vi "Func-엑셀 데이터를 그래프로 출력.vi"() -> ()   [LabVIEW 2015] (continued)
-19.24\t-17.452\n-18.3\t-19.24\t-17.442\n-18.3\t-19.23\t-17.435\n-18.3\t-19.22\t-17.427\n-18.3\t-19.22\t-17.422\n-18.3\t-19.22\t-17.417\n-18.3\t-19.21\t-17.409\n-18.3\t-19.21\t-17.403\n-18.3\t-19.2\t-17.397\n-18.3\t-19.2\t-17.384\n-18.3\t-19.19\t-17.38\n-18.3\t-19.18\t-17.376\n-18.3\t-19.17\t-17.365\n-18.3\t-19.17\t-17.361\n-18.3\t-19.16\t-17.356\n-18.3\t-19.15\t-17.347\n-18.3\t-19.15\t-17.342\n-18.3\t-19.14\t-17.333\n-18.3\t-19.14\t-17.326\n-18.3\t-19.14\t-17.316\n-18.3\t-19.14\t-17.306\n-18.3\t-19.13\t-17.302\n-18.3\t-19.12\t-17.293\n-18.3\t-19.12\t-17.285\n-18.3\t-19.11\t-17.277\n-18.3\t-19.1\t-17.278\n-18.3\t-19.1\t-17.273\n-18.3\t-19.09\t-17.261\n-18.3\t-19.08\t-17.253\n-18.3\t-19.08\t-17.249\n-18.3\t-19.07\t-17.241\n-18.3\t-19.07\t-17.228\n-18.3\t-19.06\t-17.219\n-18.3\t-19.06\t-17.211\n-18.3\t-19.05\t-17.209\n-18.3\t-19.05\t-17.198\n-18.3\t-19.04\t-17.191\n-18.3\t-19.04\t-17.187\n-18.3\t-19.03\t-17.183\n-18.3\t-19.03\t-17.173\n-18.3\t-19.02\t-17.164\n-18.3\t-19.01\t-17.159\n-18.3\t-19\t-17.15\n-18.3\t-19\t-17.142\n-18.3\t-18.99\t-17.134\n-18.3\t-18.99\t-17.129\n-18.3\t-18.99\t-17.123\n-18.3\t-18.99\t-17.114\n-18.3\t-18.98\t-17.109\n-18.3\t-18.97\t-17.102\n-18.3\t-18.97\t-17.091\n-18.3\t-18.96\t-17.084\n-18.3\t-18.95\t-17.078\n-18.3\t-18.94\t-17.068\n-18.3\t-18.94\t-17.059\n-18.3\t-18.93\t-17.053\n-18.3\t-18.93\t-17.047\n-18.3\t-18.92\t-17.04\n-18.3\t-18.92\t-17.032\n-18.3\t-18.91\t-17.025\n-18.3\t-18.91\t-17.02\n-18.3\t-18.9\t-17.014\n-18.3\t-18.9\t-17.006\n-18.3\t-18.9\t-16.998\n-18.3\t-18.9\t-16.993\n-18.3\t-18.9\t-16.983\n-18.3\t-18.89\t-16.98\n-18.3\t-18.88\t-16.971\n-18.3\t-18.87\t-16.957\n-18.3\t-18.86\t-16.95\n-18.3\t-18.86\t-16.944\n-18.3\t-18.85\t-16.934\n-18.3\t-18.84\t-16.927\n-18.3\t-18.84\t-16.92\n-18.3\t-18.84\t-16.914\n-18.3\t-18.83\t-16.914\n-18.3\t-18.83\t-16.905\n-18.3\t-18.82\t-16.9\n-18.3\t-18.82\t-16.891\n-18.3\t-18.82\t-16.887\n-18.3\t-18.81\t-16.88\n-18.3\t-18.81\t-16.871\n-18.3\t-18.8\t-16.868\n-18.3\t-18.79\t-16.857\n-18.3\t-18.79\t-16.852\n-18.3\t-18.78\t-16.845\n-18.3\t-18.78\t-16.832\n-18.3\t-18.77\t-16.824\n-18.3\t-18.76\t-16.816\n-18.3\t-18.76\t-16.809\n-18.3\t-18.75\t-16.799\n-18.3\t-18.75\t-16.791\n-18.3\t-18.75\t-16.782\n-18.3\t-18.75\t-16.776\n-18.3\t-18.74\t-16.77\n-18.3\t-18.74\t-16.761\n-18.3\t-18.74\t-16.76\n-18.3\t-18.73\t-16.756\n-18.3\t-18.72\t-16.75\n-18.3\t-18.72\t-16.744\n-18.3\t-18.71\t-16.736\n-18.3\t-18.71\t-16.73\n-18.3\t-18.7\t-16.721\n-18.3\t-18.7\t-16.713\n-18.3\t-18.69\t-16.701\n-18.3\t-18.69\t-16.693\n-18.3\t-18.68\t-16.687\n-18.3\t-18.68\t-16.675\n-18.3\t-18.67\t-16.67\n-18.3\t-18.67\t-16.664\n-18.3\t-18.67\t-16.659\n-18.3\t-18.67\t-16.653\n-18.3\t-18.66\t-16.642\n-18.3\t-18.65\t-16.634\n-18.3\t-18.65\t-16.629\n-18.3\t-18.65\t-16.62\n-18.3\t-18.64\t-16.617\n-18.3\t-18.64\t-16.611\n-18.3\t-18.63\t-16.607\n-18.3\t-18.63\t-16.601\n-18.3\t-18.62\t-16.595\n-18.3\t-18.62\t-16.587\n-18.3\t-18.62\t-16.576\n-18.3\t-18.61\t-16.569\n-18.3\t-18.61\t-16.559\n-18.3\t-18.6\t-16.552\n-18.3\t-18.6\t-16.545\n-18.3\t-18.59\t-16.534\n-18.3\t-18.59\t-16.529\n-18.3\t-18.59\t-16.523\n-18.3\t-18.59\t-16.516\n-18.3\t-18.59\t-16.508\n-18.3\t-18.59\t-16.5\n-18.3\t-18.59\t-16.493\n-18.3\t-18.58\t-16.486\n-18.3\t-18.58\t-16.478\n-18.3\t-18.58\t-16.467\n-18.3\t-18.57\t-16.461\n-18.3\t-18.56\t-16.454\n-18.3\t-18.56\t-16.446\n-18.3\t-18.55\t-16.439\n-18.3\t-18.55\t-16.431\n-18.3\t-18.54\t-16.424\n-18.3\t-18.55\t-16.419\n-18.3\t-18.54\t-16.414\n-18.3\t-18.54\t-16.404\n-18.3\t-18.53\t-16.398\n-18.3\t-18.53\t-16.395\n-18.3\t-18.53\t-16.384\n-18.3\t-18.52\t-16.379\n-18.3\t-18.52\t-16.375\n-18.3\t-18.51\t-16.366\n-18.3\t-18.51\t-16.358\n-18.3\t-18.51\t-16.35\n-18.3\t-18.51\t-16.344\n-18.3\t-18.51\t-16.331\n-18.3\t-18.51\t-16.322\n-18.3\t-18.5\t-16.316\n-18.3\t-18.5\t-16.311\n-18.3\t-18.49\t-16.304\n-18.3\t-18.49\t-16.295\n-18.3\t-18.49\t-16.293\n-18.3\t-18.49\t-16.288\n-18.3\t-18.49\t-16.28\n-18.3\t-18.49\t-16.274\n-18.3\t-18.48\t-16.265\n-18.3\t-18.48\t-16.261\n-18.3\t-18.48\t-16.254\n-18.3\t-18.48\t-16.252\n-18.3\t-18.47\t-16.242\n-18.3\t-18.47\t-16.233\n-18.3\t-18.47\t-16.224\n-18.3\t-18.46\t-16.216\n-18.3\t-18.46\t-16.209\n-18.3\t-18.46\t-16.196\n-18.3\t-18.46\t-16.188\n-18.3\t-18.45\t-16.184\n-18.3\t-18.45\t-16.177\n-18.3\t-18.45\t-16.17\n-18.3\t-18.44\t-16.164\n-18.3\t-18.44\t-16.156\n-18.3\t-18.44\t-16.149\n-18.3\t-18.44\t-16.143\n-18.3\t-18.44\t-16.132\n-18.3\t-18.44\t-16.127\n-18.3\t-18.43\t-16.121\n-18.3\t-18.43\t-16.108\n-18.3\t-18.43\t-16.102\n-18.3\t-18.43\t-16.096\n-18.3\t-18.43\t-16.089\n-18.3\t-18.43\t-16.082\n-18.3\t-18.42\t-16.074\n-18.3\t-18.42\t-16.071\n-18.3\t-18.42\t-16.064\n-18.3\t-18.42\t-16.057\n-18.3\t-18.42\t-16.052\n-18.3\t-18.42\t-16.048\n-18.3\t-18.41\t-16.043\n-18.3\t-18.4\t-16.033\n-18.3\t-18.4\t-16.026\n-18.3\t-18.4\t-16.021\n-18.3\t-18.4\t-16.01\n-18.3\t-18.4\t-16.004\n-18.3\t-18.4\t-15.996\n-18.3\t-18.4\t-15.989\n-18.3\t-18.39\t-15.983\n-18.3\t-18.39\t-15.971\n-18.3\t-18.39\t-15.962\n-18.3\t-18.39\t-15.952\n-18.3\t-18.39\t-15.949\n-18.3\t-18.39\t-15.94\n-18.3\t-18.38\t-15.936\n-18.3\t-18.38\t-15.929\n-18.3\t-18.38\t-15.921\n-18.3\t-18.37\t-15.916\n-18.3\t-18.37\t-15.909\n-18.3\t-18.37\t-15.898\n-18.3\t-18.37\t-15.892\n-18.3\t-18.37\t-15.883\n-18.3\t-18.37\t-15.876\n-18.3\t-18.37\t-15.868\n-18.3\t-18.36\t-15.858\n-18.3\t-18.36\t-15.85\n-18.3\t-18.36\t-15.841\n-18.3\t-18.36\t-15.837\n-18.3\t-18.35\t-15.831\n-18.3\t-18.35\t-15.83\n-18.3\t-18.35\t-15.822\n-18.3\t-18.35\t-15.817\n-18.3\t-18.35\t-15.812\n-18.3\t-18.35\t-15.798\n-18.3\t-18.35\t-15.792\n-18.3\t-18.35\t-15.785\n-18.3\t-18.34\t-15.777\n-18.3\t-18.34\t-15.769\n-18.3\t-18.34\t-15.763\n-18.3\t-18.34\t-15.759\n-18.3\t-18.34\t-15.752\n-18.3\t-18.33\t-15.743\n-18.3\t-18.34\t-15.735\n-18.3\t-18.33\t-15.73\n-18.3\t-18.33\t-15.723\n-18.3\t-18.33\t-15.712\n-18.3\t-18.33\t-15.707\n-18.3\t-18.33\t-15.702\n-18.3\t-18.33\t-15.695\n-18.3\t-18.33\t-15.688\n-18.3\t-18.32\t-15.685\n-18.3\t-18.32\t-15.679\n-18.3\t-18.31\t-15.67\n-18.3\t-18.31\t-15.661\n-18.3\t-18.31\t-15.653\n-18.3\t-18.31\t-15.646\n-18.3\t-18.31\t-15.639\n-18.3\t-18.31\t-15.632\n-18.3\t-18.31\t-15.63\n-18.3\t-18.31\t-15.626\n-18.3\t-18.31\t-15.619\n-18.3\t-18.31\t-15.614\n-18.3\t-18.31\t-15.607\n-18.3\t-18.31\t-15.598\n-18.3\t-18.31\t-15.589\n-18.3\t-18.31\t-15.583\n-18.3\t-18.31\t-15.57\n-18.3\t-18.31\t-15.561\n-18.3\t-18.31\t-15.553\n-18.3\t-18.31\t-15.548\n-18.3\t-18.31\t-15.544\n-18.3\t-18.31\t-15.533\n-18.3\t-18.31\t-15.533\n-18.3\t-18.31\t-15.53\n-18.3\t-18.31\t-15.518\n-18.3\t-18.31\t-15.512\n-18.3\t-18.31\t-15.504\n-18.3\t-18.31\t-15.493\n-18.3\t-18.31\t-15.485\n-18.3\t-18.31\t-15.477\n-18.3\t-18.31\t-15.467\n-18.3\t-18.31\t-15.463\n-18.3\t-18.31\t-15.458\n-18.3\t-18.31\t-15.457\n-18.3\t-18.31\t-15.448\n-18.3\t-18.31\t-15.441\n-18.3\t-18.31\t-15.433\n-18.3\t-18.31\t-15.428\n-18.3\t-18.31\t-15.422\n-18.3\t-18.31\t-15.411\n-18.3\t-18.31\t-15.407\n-18.3\t-18.31\t-15.402\n-18.3\t-18.31\t-15.395\n-18.3\t-18.31\t-15.386\n-18.3\t-18.31\t-15.38\n-18.3\t-18.31\t-15.369\n-18.3\t-18.31\t-15.359\n-18.3\t-18.31\t-15.352\n-18.3\t-18.31\t-15.343\n-18.3\t-18.31\t-15.337\n-18.3\t-18.31\t-15.33\n-18.3\t-18.31\t-15.323\n-18.3\t-18.31\t-15.32\n-18.3\t-18.29\t-15.314\n-18.3\t-18.29\t-15.307\n-18.3\t-18.29\t-15.302\n-18.3\t-18.29\t-15.293\n-18.3\t-18.29\t-15.288\n-18.3\t-18.29\t-15.279\n-18.3\t-18.29\t-15.274\n-18.3\t-18.29\t-15.266\n-18.3\t-18.29\t-15.264\n-18.3\t-18.29\t-15.257\n-18.3\t-18.29\t-15.25\n-18.3\t-18.29\t-15.243\n-18.3\t-18.29\t-15.238\n-18.3\t-18.29\t-15.228\n-18.3\t-18.29\t-15.221\n-18.3\t-18.29\t-15.216\n-18.3\t-18.29\t-15.206\n-18.3\t-18.29\t-15.203\n-18.3\t-18.29\t-15.193\n-18.3\t-18.28\t-15.185\n-18.3\t-18.29\t-15.175\n-18.3\t-18.28\t-15.172\n-18.3\t-18.29\t-15.164\n-18.3\t-18.29\t-15.159\n-18.3\t-18.29\t-15.159\n-18.3\t-18.28\t-15.148\n-18.3\t-18.28\t-15.145\n-18.3\t-18.28\t-15.133\n-18.3\t-18.28\t-15.123\n-18.3\t-18.28\t-15.115\n-18.3\t-18.28\t-15.11\n-18.3\t-18.28\t-15.108\n-18.3\t-18.28\t-15.102\n-18.3\t-18.28\t-15.095\n-18.3\t-18.28\t-15.087\n-18.3\t-18.28\t-15.081\n-18.3\t-18.28\t-15.07\n-18.3\t-18.28\t-15.064\n-18.3\t-18.28\t-15.054\n-18.3\t-18.28\t-15.05\n-18.3\t-18.28\t-15.046\n-18.3\t-18.28\t-15.041\n-18.3\t-18.28\t-15.031\n-18.3\t-18.28\t-15.022\n-18.3\t-18.28\t-15.02\n-18.3\t-18.28\t-15.012\n-18.3\t-18.28\t-15.009\n-18.3\t-18.28\t-15.002\n-18.3\t-18.28\t-14.995\n-18.3\t-18.28\t-14.986\n-18.3\t-18.28\t-14.982\n-18.3\t-18.28\t-14.973\n-18.3\t-18.28\t-14.967\n-18.3\t-18.28\t-14.961\n-18.3\t-18.28\t-14.953\n-18.3\t-18.28\t-14.95\n-18.3\t-18.28\t-14.944\n-18.3\t-18.28\t-14.931\n-18.3\t-18.28\t-14.922\n-18.3\t-18.28\t-14.918\n-18.3\t-18.28\t-14.913\n-18.3\t-18.28\t-14.908\n-18.3\t-18.28\t-14.9\n-18.3\t-18.28\t-14.896\n-18.3\t-18.28\t-14.891\n-18.3\t-18.28\t-14.885\n-18.3\t-18.28\t-14.876\n-18.3\t-18.28\t-14.871\n-18.3\t-18.28\t-14.865\n-18.3\t-18.28\t-14.86\n-18.3\t-18.28\t-14.855\n-18.3\t-18.28\t-14.848\n-18.3\t-18.28\t-14.841\n-18.3\t-18.28\t-14.833\n-18.3\t-18.28\t-14.828\n-18.3\t-18.28\t-14.818\n-18.3\t-18.28\t-14.811\n-18.3\t-18.28\t-14.806\n-18.3\t-18.28\t-14.798\n-18.3\t-18.28\t-14.791\n-18.3\t-18.28\t-14.784\n-18.3\t-18.28\t-14.776\n-18.3\t-18.28\t-14.771\n-18.3\t-18.28\t-14.764\n-18.3\t-18.28\t-14.757\n-18.3\t-18.28\t-14.753\n-18.3\t-18.28\t-14.749\n-18.3\t-18.28\t-14.745\n-18.3\t-18.28\t-14.738\n-18.3\t-18.28\t-14.728\n-18.3\t-18.28\t-14.72\n-18.3\t-18.28\t-14.713\n-18.3\t-18.28\t-14.704\n-18.3\t-18.28\t-14.696\n-18.3\t-18.28\t-14.692\n-18.3\t-18.28\t-14.685\n-18.3\t-18.28\t-14.681\n-18.3\t-18.28\t-14.676\n-18.3\t-18.28\t-14.668\n-18.3\t-18.28\t-14.661\n-18.3\t-18.28\t-14.654\n-18.3\t-18.28\t-14.646\n-18.3\t-18.28\t-14.641\n-18.3\t-18.28\t-14.634\n-18.3\t-18.28\t-14.627\n-18.3\t-18.28\t-14.622\n-18.3\t-18.28\t-14.616\n-18.3\t-18.28\t-14.607\n-18.3\t-18.28\t-14.598\n-18.3\t-18.28\t-14.593\n-18.3\t-18.28\t-14.581\n-18.3\t-18.28\t-14.573\n-18.3\t-18.28\t-14.569\n-18.3\t-18.28\t-14.56\n-18.3\t-18.28\t-14.554\n-18.3\t-18.28\t-14.552\n-18.3\t-18.28\t-14.546\n-18.3\t-18.28\t-14.545\n-18.3\t-18.28\t-14.538\n-18.3\t-18.28\t-14.533\n-18.3\t-18.28\t-14.53\n-18.3\t-18.28\t-14.52\n-18.3\t-18.28\t-14.515\n-18.3\t-18.28\t-14.51\n-18.3\t-18.28\t-14.504\n-18.3\t-18.28\t-14.496\n-18.3\t-18.28\t-14.489\n-18.3\t-18.28\t-14.486\n-18.3\t-18.28\t-14.475\n-18.3\t-18.28\t-14.466\n-18.3\t-18.28\t-14.46\n-18.3\t-18.28\t-14.457\n-18.3\t-18.28\t-14.452\n-18.3\t-18.28\t-14.446\n-18.3\t-18.28\t-14.443\n-18.3\t-18.28\t-14.436\n-18.3\t-18.28\t-14.429\n-18.3\t-18.28\t-14.423\n-18.3\t-18.28\t-14.415\n-18.3\t-18.28\t-14.404\n-18.3\t-18.28\t-14.395\n-18.3\t-18.28\t-14.392\n-18.3\t-18.28\t-14.384\n-18.3\t-18.28\t-14.374\n-18.3\t-18.27\t-14.37\n-18.3\t-18.27\t-14.369\n-18.3\t-18.27\t-14.363\n-18.3\t-18.27\t-14.356\n-18.3\t-18.27\t-14.345\n-18.3\t-18.27\t-14.342\n-18.3\t-18.27\t-14.334\n-18.3\t-18.27\t-14.323\n-18.3\t-18.28\t-14.319\n-18.3\t-18.28\t-14.311\n-18.3\t-18.28\t-14.307\n-18.3\t-18.27\t-14.302\n-18.3\t-18.27\t-14.298\n-18.3\t-18.27\t-14.29\n-18.3\t-18.27\t-14.283\n-18.3\t-18.27\t-14.277\n-18.3\t-18.27\t-14.268\n-18.3\t-18.27\t-14.261\n-18.3\t-18.27\t-14.258\n-18.3\t-18.27\t-14.252\n-18.3\t-18.27\t-14.246\n-18.3\t-18.27\t-14.243\n-18.3\t-18.27\t-14.239\n-18.3\t-18.27\t-14.233\n-18.3\t-18.27\t-14.229\n-18.3\t-18.27\t-14.22\n-18.3\t-18.27\t-14.217\n-18.3\t-18.27\t-14.213\n-18.3\t-18.27\t-14.204\n-18.3\t-18.27\t-14.199\n-18.3\t-18.27\t-14.191\n-18.3\t-18.27\t-14.182\n-18.3\t-18.27\t-14.174\n-18.3\t-18.27\t-14.168\n-18.3\t-18.27\t-14.16\n-18.3\t-18.27\t-14.156\n-18.3\t-18.27\t-14.15\n-18.3\t-18.27\t-14.144\n-18.3\t-18.27\t-14.142\n-18.3\t-18.27\t-14.138\n-18.3\t-18.27\t-14.131\n-18.3\t-18.27\t-14.125\n-18.3\t-18.27\t-14.121\n-18.3\t-18.27\t-14.112\n-18.3\t-18.27\t-14.103\n-18.3\t-18.27\t-14.096\n-18.3\t-18.27\t-14.088\n-18.3\t-18.27\t-14.085\n-18.3\t-18.27\t-14.077\n-18.3\t-18.27\t-14.074\n-18.3\t-18.27\t-14.071\n-18.3\t-18.27\t-14.063\n-18.3\t-18.27\t-14.055\n-18.3\t-18.27\t-14.05\n-18.3\t-18.27\t-14.045\n-18.3\t-18.27\t-14.035\n-18.3\t-18.27\t-14.029\n-18.3\t-18.27\t-14.027\n-18.3\t-18.27\t-14.018\n-18.3\t-18.27\t-14.011\n-18.3\t-18.27\t-14.01\n-18.3\t-18.27\t-14.003\n-18.3\t-18.27\t-13.998\n-18.3\t-18.27\t-13.993\n-18.3\t-18.27\t-13.99\n-18.3\t-18.27\t-13.981\n-18.3\t-18.27\t-13.973\n-18.3\t-18.27\t-13.964\n-18.3\t-18.27\t-13.959\n-18.3\t-18.27\t-13.954\n-18.3\t-18.27\t-13.946\n-18.3\t-18.27\t-13.946\n-18.3\t-18.27\t-13.942\n-18.3\t-18.27\t-13.937\n-18.3\t-18.27\t-13.93\n-18.3\t-18.27\t-13.925\n-18.3\t-18.27\t-13.919\n-18.3\t-18.27\t-13.913\n-18.3\t-18.27\t-13.902\n-18.3\t-18.27\t-13.898\n-18.3\t-18.27\t-13.894\n-18.3\t-18.27\t-13.888\n-18.3\t-18.27\t-13.88\n-18.3\t-18.27\t-13.872\n-18.3\t-18.27\t-13.862\n-18.3\t-18.27\t-13.856\n-18.3\t-18.27\t-13.851\n-18.3\t-18.27\t-13.844\n-18.3\t-18.27\t-13.839\n-18.3\t-18.27\t-13.833\n-18.3\t-18.27\t-13.831\n-18.3\t-18.27\t-13.827\n-18.3\t-18.27\t-13.822\n-18.3\t-18.27\t-13.816\n-18.3\t-18.27\t-13.816\n-18.3\t-18.27\t-13.811\n-18.3\t-18.27\t-13.803\n-18.3\t-18.27\t-13.8\n-18.3\t-18.27\t-13.792\n-18.3\t-18.27\t-13.783\n-18.3\t-18.27\t-13.774\n-18.3\t-18.27\t-13.767\n-18.3\t-18.27\t-13.756\n-18.3\t-18.28\t-13.747\n-18.3\t-18.28\t-13.744\n-18.3\t-18.28\t-13.739\n-18.3\t-18.28\t-13.735\n-18.3\t-18.28\t-13.732\n-18.3\t-18.28\t-13.726\n-18.3\t-18.28\t-13.722\n-18.3\t-18.28\t-13.714\n-18.3\t-18.28\t-13.707\n-18.3\t-18.28\t-13.702\n-18.3\t-18.28\t-13.696\n-18.3\t-18.28\t-13.694\n-18.3\t-18.28\t-13.687\n-18.3\t-18.28\t-13.684\n-18.3\t-18.28\t-13.678\n-18.3\t-18.28\t-13.671\n-18.3\t-18.28\t-13.667\n-18.3\t-18.28\t-13.659\n-18.3\t-18.28\t-13.655\n-18.3\t-18.28\t-13.65\n-18.3\t-18.28\t-13.642\n-18.3\t-18.28\t-13.637\n-18.3\t-18.28\t-13.634\n-18.3\t-18.28\t-13.627\n-18.3\t-18.28\t-13.62\n-18.3\t-18.28\t-13.616\n-18.3\t-18.28\t-13.612\n-18.3\t-18.28\t-13.607\n-18.3\t-18.28\t-13.598\n-18.3\t-18.28\t-13.592\n-18.3\t-18.28\t-13.59\n-18.3\t-18.28\t-13.584\n-18.3\t-18.28\t-13.576\n-18.3\t-18.28\t-13.568\n-18.3\t-18.28\t-13.564\n-18.3\t-18.28\t-13.556\n-18.3\t-18.28\t-13.548\n-18.3\t-18.28\t-13.54\n-18.3\t-18.28\t-13.534\n-18.3\t-18.28\t-13.534\n-18.3\t-18.28\t-13.526\n-18.3\t-18.28\t-13.523\n-18.3\t-18.28\t-13.518\n-18.3\t-18.28\t-13.511\n-18.3\t-18.28\t-13.506\n-18.3\t-18.28\t-13.498\n-18.3\t-18.28\t-13.492\n-18.3\t-18.28\t-13.486\n-18.3\t-18.28\t-13.48\n-18.3\t-18.28\t-13.476\n-18.3\t-18.28\t-13.472\n-18.3\t-18.28\t-13.468\n-18.3\t-18.28\t-13.463\n-18.3\t-18.28\t-13.459\n-18.3\t-18.28\t-13.454\n-18.3\t-18.28\t-13.447\n-18.3\t-18.28\t-13.442\n-18.3\t-18.28\t-13.437\n-18.3\t-18.28\t-13.43\n-18.3\t-18.28\t-13.425\n-18.3\t-18.28\t-13.42\n-18.3\t-18.28\t-13.413\n-18.3\t-18.28\t-13.407\n-18.3\t-18.28\t-13.402\n-18.3\t-18.28\t-13.394\n-18.3\t-18.28\t-13.389\n-18.3\t-18.28\t-13.386\n-18.3\t-18.28\t-13.378\n-18.3\t-18.28\t-13.375\n-18.3\t-18.29\t-13.37\n-18.3\t-18.29\t-13.365\n-18.3\t-18.29\t-13.361\n-18.3\t-18.29\t-13.356\n-18.3\t-18.29\t-13.348\n-18.3\t-18.29\t-13.343\n-18.3\t-18.29\t-13.341\n-18.3\t-18.29\t-13.333\n-18.3\t-18.29\t-13.329\n-18.3\t-18.29\t-13.322\n-18.3\t-18.29\t-13.318\n-18.3\t-18.29\t-13.313\n-18.3\t-18.29\t-13.307\n-18.3\t-18.29\t-13.302\n-18.3\t-18.29\t-13.299\n-18.3\t-18.29\t-13.296\n-18.3\t-18.29\t-13.288\n-18.3\t-18.29\t-13.284\n-18.3\t-18.29\t-13.276\n-18.3\t-18.29\t-13.27\n-18.3\t-18.29\t-13.264\n-18.3\t-18.29\t-13.257\n-18.3\t-18.29\t-13.256\n-18.3\t-18.29\t-13.25\n-18.3\t-18.29\t-13.245\n-18.3\t-18.29\t-13.242\n-18.3\t-18.29\t-13.235\n-18.3\t-18.29\t-13.231\n-18.3\t-18.29\t-13.224\n-18.3\t-18.29\t-13.219\n-18.3\t-18.29\t-13.21\n-18.3\t-18.29\t-13.204\n-18.3\t-18.31\t-13.202\n-18.3\t-18.31\t-13.196\n-18.3\t-18.31\t-13.192\n-18.3\t-18.31\t-13.187\n-18.3\t-18.31\t-13.183\n-18.3\t-18.31\t-13.178\n-18.3\t-18.31\t-13.173\n-18.3\t-18.31\t-13.168\n-18.3\t-18.31\t-13.163\n-18.3\t-18.31\t-13.161\n-18.3\t-18.31\t-13.155\n-18.3\t-18.31\t-13.151\n-18.3\t-18.31\t-13.144\n-18.3\t-18.31\t-13.139\n-18.3\t-18.31\t-13.135\n-18.3\t-18.31\t-13.129\n-18.3\t-18.31\t-13.119\n-18.3\t-18.31\t-13.114\n-18.3\t-18.31\t-13.111\n-18.3\t-18.31\t-13.102\n-18.3\t-18.29\t-13.096\n-18.3\t-18.29\t-13.093\n-18.3\t-18.29\t-13.089\n-18.3\t-18.29\t-13.087\n-18.3\t-18.29\t-13.081\n-18.3\t-18.31\t-13.079\n-18.3\t-18.31\t-13.075\n-18.3\t-18.31\t-13.07\n-18.3\t-18.31\t-13.065\n-18.3\t-18.31\t-13.058\n-18.3\t-18.31\t-13.052\n-18.3\t-18.31\t-13.041\n-18.3\t-18.31\t-13.038\n-18.3\t-18.31\t-13.032\n-18.3\t-18.31\t-13.026\n-18.3\t-18.31\t-13.022\n-18.3\t-18.31\t-13.019\n-18.3\t-18.31\t-13.016\n-18.3\t-18.31\t-13.009\n-18.3\t-18.31\t-13.005\n-18.3\t-18.31\t-13.001\n-18.3\t-18.31\t-12.997\n-18.3\t-18.31\t-12.991\n-18.3\t-18.31\t-12.982\n-18.3\t-18.31\t-12.979\n-18.3\t-18.31\t-12.97\n-18.3\t-18.31\t-12.966\n-18.3\t-18.31\t-12.961\n-18.3\t-18.31\t-12.959\n-18.3\t-18.31\t-12.954\n-18.3\t-18.31\t-12.948\n-18.3\t-18.31\t-12.941\n-18.3\t-18.31\t-12.936\n-18.3\t-18.31\t-12.932\n-18.3\t-18.31\t-12.922\n-18.3\t-18.31\t-12.918\n-18.3\t-18.31\t-12.914\n-18.3\t-18.31\t-12.908\n-18.3\t-18.31\t-12.904\n-18.3\t-18.31\t-12.9\n-18.3\t-18.31\t-12.893\n-18.3\t-18.31\t-12.891\n-18.3\t-18.31\t-12.888\n-18.3\t-18.31\t-12.886\n-18.3\t-18.31\t-12.88\n-18.3\t-18.31\t-12.875\n-18.3\t-18.31\t-12.869\n-18.3\t-18.31\t-12.864\n-18.3\t-18.31\t-12.858\n-18.3\t-18.31\t-12.852\n-18.3\t-18.31\t-12.846\n-18.3\t-18.31\t-12.841\n-18.3\t-18.31\t-12.835\n-18.3\t-18.31\t-12.828\n-18.3\t-18.31\t-12.827\n-18.3\t-18.31\t-12.818\n-18.3\t-18.31\t-12.818\n-18.3\t-18.31\t-12.818\n-18.3\t-18.31\t-12.816\n-18.3\t-18.31\t-12.813\n-18.3\t-18.31\t-12.808\n-18.3\t-18.31\t-12.806\n-18.3\t-18.31\t-12.796\n-18.3\t-18.31\t-12.79\n-18.3\t-18.31\t-12.784\n-18.3\t-18.31\t-12.782\n-18.3\t-18.31\t-12.776\n-18.3\t-18.31\t-12.77\n-18.3\t-18.31\t-12.769\n-18.3\t-18.31\t-12.765\n-18.3\t-18.31\t-12.758\n-18.3\t-18.31\t-12.754\n-18.3\t-18.31\t-12.748\n-18.3\t-18.31\t-12.743\n-18.3\t-18.31\t-12.736\n-18.3\t-18.31\t-12.73\n-18.3\t-18.31\t-12.731\n-18.3\t-18.31\t-12.724\n-18.3\t-18.31\t-12.719\n-18.3\t-18.31\t-12.713\n-18.3\t-18.31\t-12.712\n-18.3\t-18.31\t-12.705\n-18.3\t-18.31\t-12.699\n-18.3\t-18.31\t-12.696\n-18.3\t-18.31\t-12.689\n-18.3\t-18.31\t-12.689\n-18.3\t-18.31\t-12.685\n-18.3\t-18.31\t-12.68\n-18.3\t-18.31\t-12.675\n-18.3\t-18.31\t-12.671\n-18.3\t-18.31\t-12.668\n-18.3\t-18.31\t-12.665\n-18.3\t-18.31\t-12.661\n-18.3\t-18.31\t-12.654\n-18.3\t-18.31\t-12.645\n-18.3\t-18.31\t-12.642\n-18.3\t-18.31\t-12.634\n-18.3\t-18.31\t-12.629\n-18.3\t-18.31\t-12.624\n-18.3\t-18.31\t-12.616\n-18.3\t-18.31\t-12.617\n-18.3\t-18.31\t-12.613\n-18.3\t-18.31\t-12.606\n-18.3\t-18.31\t-12.598\n-18.3\t-18.31\t-12.593\n-18.3\t-18.31\t-12.589\n-18.3\t-18.31\t-12.584\n-18.3\t-18.31\t-12.579\n-18.3\t-18.31\t-12.574\n-18.3\t-18.31\t-12.572\n-18.3\t-18.31\t-12.567\n-18.3\t-18.31\t-12.568\n-18.3\t-18.31\t-12.564\n-18.3\t-18.31\t-12.561\n-18.3\t-18.31\t-12.555\n-18.3\t-18.31\t-12.552\n-18.3\t-18.31\t-12.546\n-18.3\t-18.31\t-12.537\n-18.3\t-18.31\t-12.532\n-18.3\t-18.31\t-12.527\n-18.3\t-18.31\t-12.522\n-18.3\t-18.31\t-12.518\n-18.3\t-18.31\t-12.517\n-18.3\t-18.31\t-12.51\n-18.3\t-18.31\t-12.507\n-18.3\t-18.31\t-12.504\n-18.3\t-18.31\t-12.498\n-18.3\t-18.31\t-12.491\n-18.3\t-18.31\t-12.489\n-18.3\t-18.31\t-12.484\n-18.3\t-18.31\t-12.479\n-18.3\t-18.31\t-12.474\n-18.3\t-18.31\t-12.468\n-18.3\t-18.31\t-12.465\n-18.3\t-18.31\t-12.459\n-18.3\t-18.31\t-12.454\n-18.3\t-18.31\t-12.448\n-18.3\t-18.31\t-12.446\n-18.3\t-18.31\t-12.442\n-18.3\t-18.31\t-12.438\n-18.3\t-18.31\t-12.434\n-18.3\t-18.31\t-12.426\n-18.3\t-18.31\t-12.423\n-18.3\t-18.31\t-12.418\n-18.3\t-18.31\t-12.415\n-18.3\t-18.31\t-12.413\n-18.3\t-18.31\t-12.413\n-18.3\t-18.31\t-12.409\n-18.3\t-18.31\t-12.408\n-18.3\t-18.31\t-12.404\n-18.3\t-18.31\t-12.396\n-18.3\t-18.31\t-12.39\n-18.3\t-18.31\t-12.385\n-18.3\t-18.31\t-12.385\n-18.3\t-18.31\t-12.38\n-18.3\t-18.31\t-12.376\n-18.3\t-18.31\t-12.373\n-18.3\t-18.31\t-12.37\n-18.3\t-18.31\t-12.366\n-18.3\t-18.31\t-12.36\n-18.3\t-18.31\t-12.354\n-18.3\t-18.31\t-12.351\n-18.3\t-18.31\t-12.348\n-18.3\t-18.31\t-12.345\n-18.3\t-18.31\t-12.34\n-18.3\t-18.31\t-12.334\n-18.3\t-18.31\t-12.333\n-18.3\t-18.31\t-12.328\n-18.3\t-18.31\t-12.32\n-18.3\t-18.31\t-12.314\n-18.3\t-18.31\t
